vi "Do Request.vi"(8 "error in (no error)":errorcluster, 9 "Body (Empty)":string, 10 "Client Data":T1={"HTTP Method"=enum."GET", "URL Path"="", "Access ID"="PqVr/ifkAQh+lVrdPIykXlFvg12GhhQFR8H9cUhphgg=", "Secret ID"="pTe9HRlQuMfJxAG6QCGq7UvoUpJzAzWGKy5SbZ+roSU="}, 11 "URL":string) -> (0 "error out":errorcluster, 2 "Response Body":string)   [LabVIEW 2020, in "WS Admin.lvlib"]
uses:
  WS Admin.lvlib
  Client Data.ctl
  HTTP Method.ctl
  <vilib>/httpClient/POSTBuffer.vi
  <vilib>/httpClient/PUTBuffer.vi
  <vilib>/regexp/Match Regular Expression.xnode
  <vilib>/httpClient/LabVIEWHTTPClient.lvlib
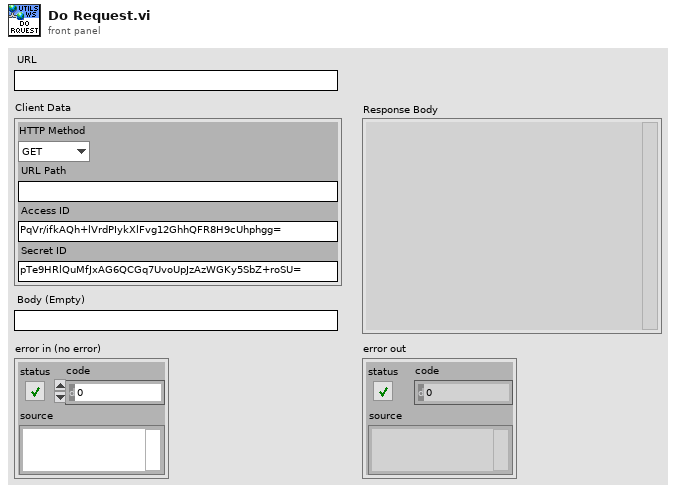
[diagram p1: front panel]
types:
  T1 = typedef "WS Admin.lvlib/Client Data.ctl" = cluster{"HTTP Method":T2, "URL Path":string, "Access ID":string, "Secret ID":string}
  T2 = typedef "WS Admin.lvlib/HTTP Method.ctl" = enum16{"GET", "POST", "PUT", "DELETE"}
  T3 = typedef "LabVIEWHTTPClient.lvlib/ClientHandle.ctl" = refnum<k1>
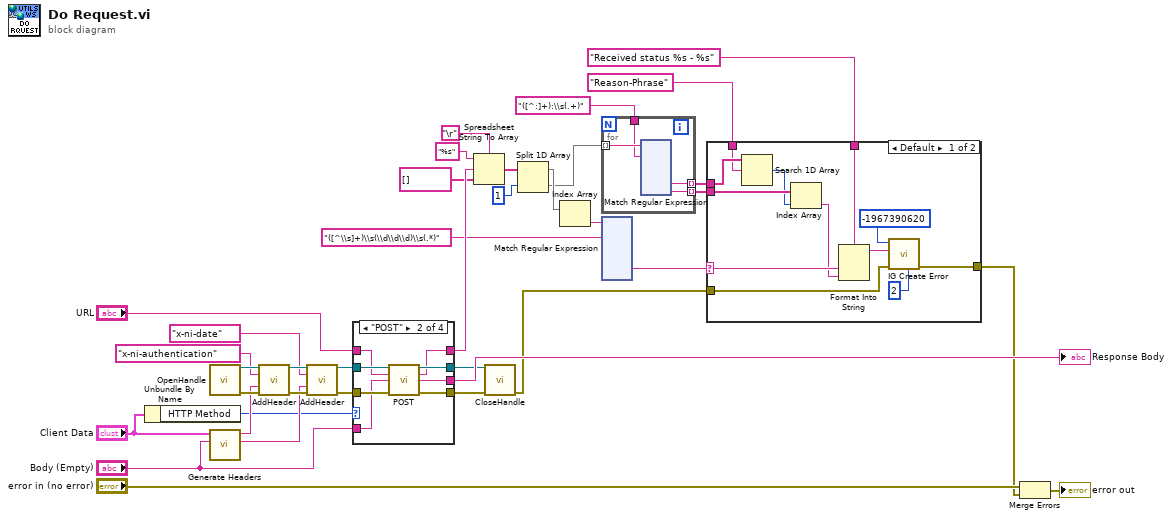
[diagram p0: block diagram]
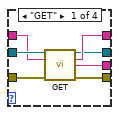
[diagram p3: hidden frame]
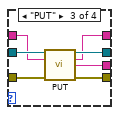
[diagram p4: hidden frame]
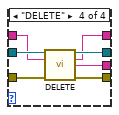
[diagram p5: hidden frame]
diagram:
  n1 = Unbundle By Name("Client Data") -> ("HTTP Method"=w26:T2)
  n2 = call <vilib>:"OpenHandle.vi"() -> ("client handle out"=w36:T3, "error out"=w37:errorcluster)  [unwired: 14 in]
  n3 = call "Generate Headers.vi"("Content Body (Empty)"="Body (Empty)", "Client Data"="Client Data") -> ("x-ni-date"=w31:string, "x-ni-authentication"=w34:string)  [unwired: 8 in]
  n4 = call <vilib>:"AddHeader.vi"("client handle"=w36, "header"="x-ni-authentication", "value"=w34, "error in (no error)"=w37) -> ("client handle out"=w33:T3, "error out"=w32:errorcluster)  [unwired: 10 in]
  n5 = call <vilib>:"AddHeader.vi"("client handle"=w33, "header"="x-ni-date", "value"=w31, "error in (no error)"=w32) -> ("client handle out"=w28:T3, "error out"=w27:errorcluster)  [unwired: 10 in]
  n6 = case shown="\"POST\"" w26 {
    tunnel: w28 -> [w44 w52 w59 w66]
    tunnel: w27 -> [w43 w51 w58 w65]
    tunnel: "URL" -> [w42 w50 w57 w64]
    tunnel: [w41 w48 w55 w62] -> w20
    tunnel: [w40 w47 w54 w61] -> w23
    tunnel: [w39 w49 w56 w63] -> w16
    tunnel: [w38 w46 w53 w60] -> w15
    tunnel: "Body (Empty)" -> [_ w45 _ _]
    frame "GET" {
      n7 = call <vilib>:"GET.vi"("client handle"=w44, "url"=w42, "error in (no error)"=w43) -> ("client handle out"=w39:T3, "headers"=w41:string, "body"=w40:string, "error out"=w38:errorcluster)  [unwired: 9 in]
    }
    frame "POST" {
      n8 = call-poly <vilib>:"POST.vi"("client handle"=w52, "url"=w50, "buffer"=w45, "error in (no error)"=w51) -> ("client handle out"=w49:T3, "headers"=w48:string, "body"=w47:string, "error out"=w46:errorcluster)  [unwired: 8 in]
    }
    frame "PUT" {
      n9 = call-poly <vilib>:"PUT.vi"("client handle"=w59, "url"=w57, "error in (no error)"=w58) -> ("client handle out"=w56:T3, "headers"=w55:string, "body"=w54:string, "error out"=w53:errorcluster)  [unwired: 9 in]
    }
    frame "DELETE" {
      n10 = call <vilib>:"DELETE.vi"("client handle"=w66, "url"=w64, "error in (no error)"=w65) -> ("client handle out"=w63:T3, "headers"=w62:string, "body"=w61:string, "error out"=w60:errorcluster)  [unwired: 9 in]
    }
  }
  "Response Body" <- w23
  n11 = Spreadsheet String To Array(delimiter (Tab)="\r", format string="%s", spreadsheet string=w20, array type (2D Dbl)=string[] []) -> (array=w14:string[])
  n12 = call <vilib>:"CloseHandle.vi"("client handle"=w16, "error in (no error)"=w15) -> ("error out"=w3:errorcluster)  [unwired: 13 in]
  n13 = Split 1D Array(array=w14, index=1 ("length")) -> (first subarray=w10:string[], second subarray=w1:string[])
  n14 = Index Array(array=w10) -> (element=w12:string)  [unwired: 1 in]
  n15 = for {
    tunnel: w1 -> [w70] mode=indexing
    tunnel: "([^:]+):\\s(.+)" ("regular expression") -> [w69]
    tunnel: [w68] -> w7 mode=indexing
    tunnel: [w67] -> w6 mode=indexing
    n16 = xnode "Match Regular Expression"("input string"=w70, "regular expression"=w69) -> ("submatch 1"=w68:string, "submatch 2"=w67:string)  [unwired: 4 in, 5 out]
  }
  n17 = xnode "Match Regular Expression"("input string"=w12, "regular expression"="([^\\s]+)\\s(\\d\\d\\d)\\s(.*)") -> ("submatch 2"=w8:string)  [unwired: 4 in, 7 out]
  n18 = case shown="Default" w8 {
    selector: w8 -> [w197 _]
    tunnel: w7 -> [w199 _]
    tunnel: w6 -> [w195 _]
    tunnel: "Received status %s - %s" -> [w198 _]
    tunnel: "Reason-Phrase" -> [w196 _]
    tunnel: w3 -> [w190 _]
    tunnel: [w189 _] -> w2
    frame Default {
      n19 = Search 1D Array(1D array=w199, element=w196) -> (index of element=w194:i32)  [unwired: 1 in]
      n20 = Index Array(array=w195, index=w194) -> (element=w193:string)
      n21 = Format Into String(format string=w198, w197, w193) -> (resulting string=w192:string)  [unwired: 2 in, 1 out]
      n22 = call "IG Create Error.vi"("Skip Call Stack (1)"=2, "error in (no error)"=w190, "Message (\"\")"=w192, "Code"=-1967390620) -> ("error out"=w189:errorcluster)  [unwired: 7 in]
    }
    frame "200" {
    }
  }
  n23 = Merge Errors("error in (no error)", w2) -> (→"error out":errorcluster)
